vi "MH_T2 Read Acq Q_TT.vi"() -> ()   [LabVIEW 2019]
uses:
  <userlib>/MultiHarp150/T2Lib/MH_T2DeltaQMessage.ctl
  <userlib>/MultiHarp150/T2Lib/MH_T2QMessage.ctl
panel:
  out "TraceSize":u64
  in  "Bin size(ns)":u64
  in  "Tracelenght(s)":u64=16
  out "Done":bool
  out "TotalRec":i32
  out "TotalTime":u32
  in  "stop":bool
  out "sortie d'erreur":errorcluster caption="ErrorOut"
  out "RollOver":bool
  in  "Save Data":bool
  in  "StopCh":u32=2
  in  "StartCh":u32=1
  out "DeltaT":u32[](array[numeric])
  out "nActual":i32[](array[numeric])
  out "En Attente":i32[](array[numeric])
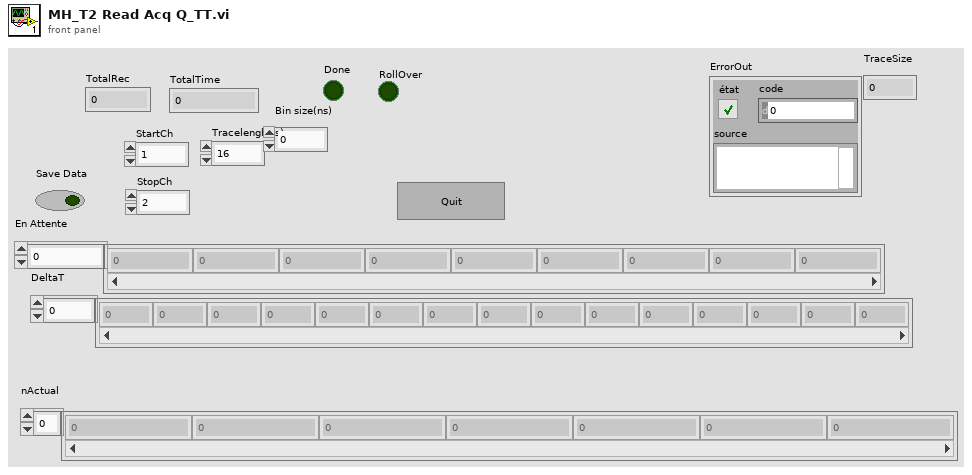
[diagram p1: front panel]
types:
  T1 = typedef "MH_T2DeltaQMessage.ctl" = cluster{"Message":string, "buffer":i32[], "Code":i32, "nactual":i32}
  T2 = typedef "MH_T2QMessage.ctl" = cluster{"Message":string, "buffer":u32[], "Code":i32, "nactual":i32}
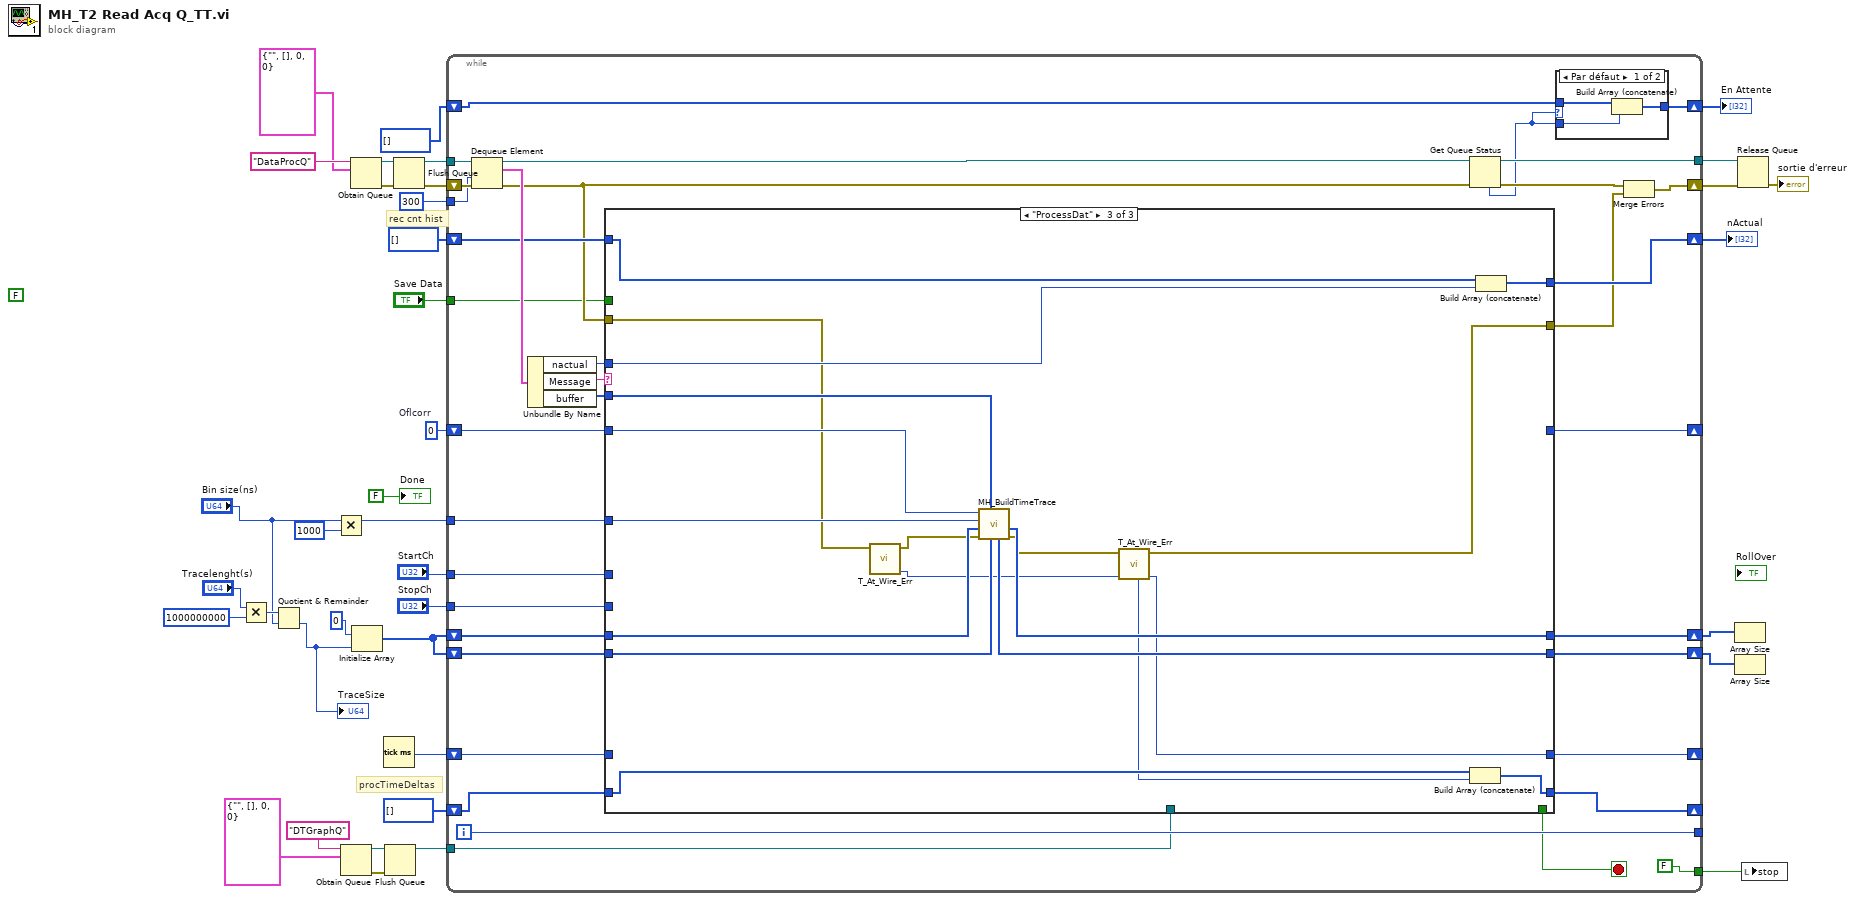
[diagram p0: block diagram]
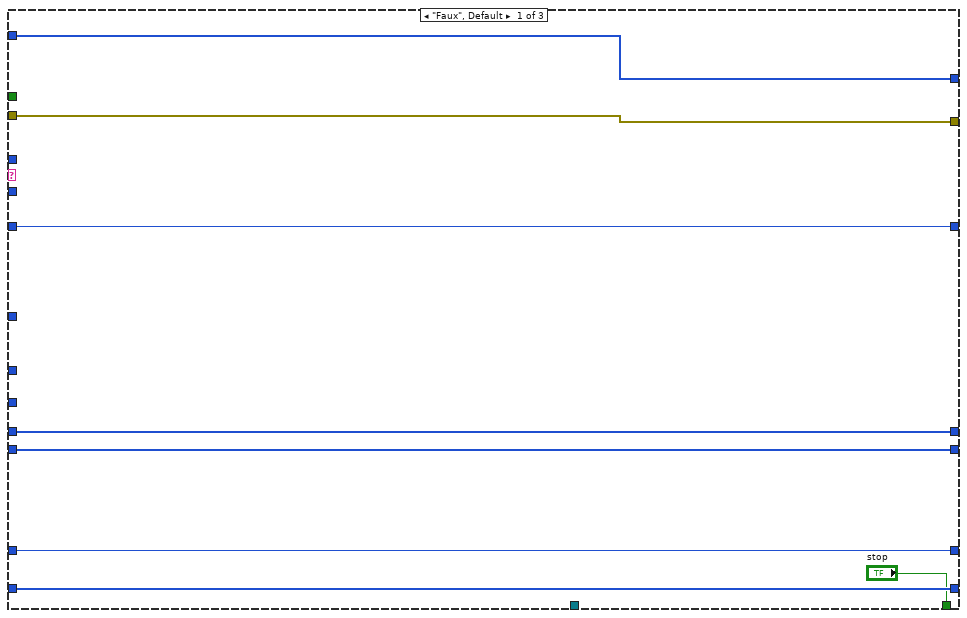
[diagram p2: hidden frame]
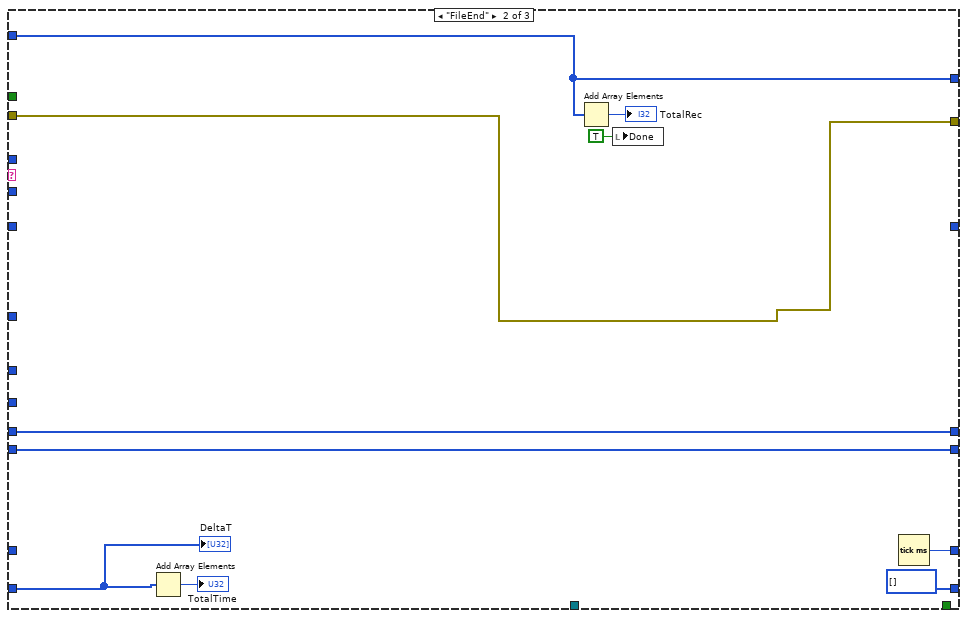
[diagram p3: hidden frame]
diagram:
  (unwired) FALSE
  w36 = u64 0  # Oflcorr
  # "procTimeDeltas"
  # "rec cnt hist"
  n1 = Multiply(x="Tracelenght(s)", y=u64 1000000000) -> (x*y=w6:u64)
  n2 = Quotient & Remainder(x=w6, y="Bin size(ns)") -> (floor(x/y)=w3:u64)  [unwired: 1 out]
  "TraceSize" <- w3
  n3 = Multiply(x="Bin size(ns)", y=u64 1000) -> (x*y=w2:u64)
  n4 = Obtain Queue(name (unnamed)="DTGraphQ" ("nom (aucun)"), element data type=T1 {"Message"="", "buffer"=[], "Code"=0, "nactual"=0} ("ClassQueue")) -> (queue out=w14:refnum<queue>, error out=w15:errorcluster)  [unwired: 3 in, 1 out]
  n5 = Obtain Queue(name (unnamed)="DataProcQ" ("nom (aucun)"), element data type=T2 {"Message"="", "buffer"=[], "Code"=0, "nactual"=0} ("ClassQueue")) -> (queue out=w19:refnum<queue>, error out=w16:errorcluster)  [unwired: 3 in, 1 out]
  n6 = Initialize Array(u64 0 ("truetime"), w3) -> (w11:u64[])
  n7 = Tick Count (ms)() -> (millisecond timer value=w32:u32)
  n8 = Flush Queue(queue=w14, error in (no error)=w15) -> (queue out=w21:refnum<queue>)  [unwired: 2 out]
  n9 = Flush Queue(queue=w19, error in (no error)=w16) -> (queue out=w18:refnum<queue>, error out=w17:errorcluster)  [unwired: 1 out]
  n10 = while {
    tunnel: w18 -> [w73]
    shift-right: [w54] -> w35
    shift-left: w17 -> [w74]
    shift-right: [w71] -> _
    shift-left: w36 -> [w72]
    tunnel: [w68] -> _
    tunnel: [w64] -> w34
    shift-right: [w62] -> _
    shift-left: w32 -> [w63]
    shift-right: [w60] -> _
    shift-left: u32[] [] ("DeltaT") -> [w61]
    shift-right: [w58] -> w29
    shift-left: i32[] [] ("DeltaT") -> [w59]
    shift-right: [w57] -> w33
    shift-left: i32[] [] ("DeltaT") -> [w56]
    tunnel: "Save Data" -> [w53]
    shift-right: [w50] -> w9
    shift-left: w11 -> [w52]
    tunnel: "StopCh" -> [w51]
    tunnel: 300 ("timeout en ms (-1)") -> [w49]
    tunnel: w21 -> [w47]
    tunnel: [FALSE] -> w13
    shift-right: [w41] -> w8
    shift-left: w11 -> [w42]
    tunnel: "StartCh" -> [w40]
    tunnel: w2 -> [w39]
    i -> [w68]
    stop <- w45 stop-if-true
    n11 = Dequeue Element(queue=w73, timeout in ms (-1)=w49, error in (no error)=w74) -> (queue out=w66:refnum<queue>, element=w70:T2, error out=w55:errorcluster)  [unwired: 1 out]
    n12 = Unbundle By Name(w70) -> ("nactual"=w48:i32, "Message"=w67:string, "buffer"=w69:u32[])
    n13 = case shown="\"ProcessDat\"" w67 {
      tunnel: w72 -> [w82 _ w102]
      tunnel: [w82 _ _] -> w71
      tunnel: w69 -> [_ _ w111]
      tunnel: w63 -> [w81 _ _]
      tunnel: [w80 u32[] [] ("DeltaT") w95] -> w60
      tunnel: [w81 w91 w96] -> w62
      tunnel: w61 -> [w80 w89 w94]
      tunnel: w59 -> [w79 w87 w104]
      tunnel: [w79 w87 w105] -> w58
      tunnel: w55 -> [w77 w83 w101]
      tunnel: w53 -> [_ _ _]
      tunnel: w52 -> [w78 w92 w109]
      tunnel: w51 -> [_ _ _]
      tunnel: [w78 w92 w107] -> w50
      tunnel: w48 -> [_ _ w103]
      tunnel: w47 -> [_ _ _]
      tunnel: [w77 w83 w98] -> w46
      tunnel: ["stop" _ _] -> w45
      tunnel: w42 -> [w75 w84 w108]
      tunnel: [w75 w84 w106] -> w41
      tunnel: w40 -> [_ _ _]
      tunnel: w39 -> [_ _ w110]
      frame "Faux", Default {
      }
      frame "FileEnd" {
        n14 = Add Array Elements(numeric array=w89) -> (sum=→"TotalTime":u32)
        n15 = Add Array Elements(numeric array=w87) -> (sum=→"TotalRec":i32)
        n16 = local write "Done"(TRUE ("Done")) -> ()
        n17 = Tick Count (ms)() -> (millisecond timer value=w91:u32)
        "DeltaT" <- w89
      }
      frame "ProcessDat" {
        n18 = call <userlib>:"T_At_Wire_Err.vi"("error in (no error)"=w101) -> ("Clock(ms)"=w97:u32, "error out"=w100:errorcluster)  [unwired: 8 in, 1 out]
        n19 = call <userlib>:"MH_BuildTimeTrace.vi"("Trace2_In"=w108, "rawbits"=w111, "error in (no error)"=w100, "Trace1_In"=w109, "Bin size(ps)"=w110, "oflcorr_in"=w102) -> ("error out"=w99:errorcluster, "Trace1_Out"=w107:u64[], "Trace2_Out"=w106:u64[])  [unwired: 2 in, 1 out]
        n20 = call <userlib>:"T_At_Wire_Err.vi"("InitClock(ms)"=w97, "error in (no error)"=w99) -> ("Clock(ms)"=w96:u32, "error out"=w98:errorcluster, "Delta(ms)"=w93:u32)  [unwired: 7 in]
        n21 = Build Array (concatenate)(w94, w93) -> (w95:u32[])
        n22 = Build Array (concatenate)(w104, w103) -> (w105:i32[])
      }
    }
    n23 = Get Queue Status(queue=w66, error in (no error)=w55) -> (queue out=w64:refnum<queue>, error out=w65:errorcluster, # elements in queue=w43:i32)  [unwired: 1 in, 5 out]
    n24 = case shown="Par défaut" w43 {
      tunnel: w43 -> [w114 _]
      tunnel: [w113 w115] -> w57
      tunnel: w56 -> [w112 w115]
      frame Default {
        n25 = Build Array (concatenate)(w112, w114) -> (w113:i32[])
      }
      frame 0 {
      }
    }
    n26 = Merge Errors(w65, w46) -> (w54:errorcluster)
  }
  "En Attente" <- w33
  "nActual" <- w29
  n27 = Array Size(array=w9) -> ()  [unwired: 1 out]
  n28 = Array Size(array=w8) -> ()  [unwired: 1 out]
  n29 = Release Queue(queue=w34, error in (no error)=w35) -> (error out=→"sortie d'erreur":errorcluster)  [unwired: 1 in, 2 out]
  n30 = local write "stop"(w13) -> ()
  "Done" <- FALSE
